vi "setStepNLoopParams.vi"(0 "Controller in":refnum<class "_Controller.lvclass">, 2 "axis (only applicable to multi-axis applications)":T3, 3 "set_params?":T2, 4 "step_n_params":T1, 5 "error in (no error)":errorcluster) -> (14 "Controller out":refnum<class "_Controller.lvclass">, 17 "success?":bool, 18 "response":string, 19 "error out":errorcluster)   [LabVIEW 2020, in "classes.lvlib" / "_Controller.lvclass"]
doc: "Use this VI to set the Step N Loop parameters to the referenced device at the specified index. For single axis applications, the axis input need not be specified.\n\nThere are two key cluster inputs to this VI: \"set_params?\" and \"set_n_params\". \n\n<B>step_n_params</B> allows the user to set the Step N Paramters if his/her choosing (minus the \"enabled\" status, which is handled via the Enable Step N Loop and Disable Step N Loop action VIs). \n<B>set_params?</B> contains boolean values that correspond to each settable parameter.\n\nIf the User wishes to only set the step_N_loop_ratio value to .75 while leaving all other parameters untouched, simply fill in the step_N_loop_ratio entry in the step_n_params cluster and set ONLY the \"set_ratio?\" boolean to TRUE in the \"set_params?' cluster.\n\nProduced By:\n\n<B>Kod Integrations, LLC</B>\n4835 Marianne Drive\nMount Airy, MD 21771\nhttp://www.kodintegrations.com\nemail: info@kodintegrations.com\nphone: (240) 687-1288"
uses:
  _Controller.lvclass
  common/controls/axis.ctl
  common/controls/step_n_loop_params_write_logic.ctl
  common/controls/step_n_params.ctl
  libraries/common.lvlib
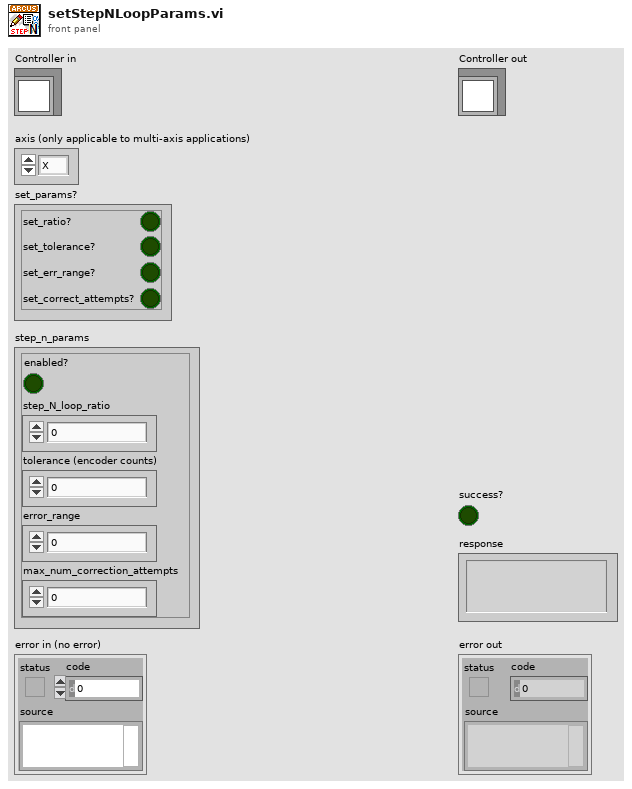
[diagram p1: front panel]
types:
  T1 = typedef "common.lvlib/step_n_params.ctl" = cluster{"step_N_loop_ratio":dbl, "tolerance (encoder counts)":u32, "error_range":i32, "max_num_correction_attempts":i32, "enabled?":bool}
  T2 = typedef "common.lvlib/step_n_loop_params_write_logic.ctl" = cluster{"set_ratio?":bool, "set_tolerance?":bool, "set_err_range?":bool, "set_correct_attempts?":bool}
  T3 = typedef "common.lvlib/axis.ctl" = enum16{"X", "Y", "Z", "U"}
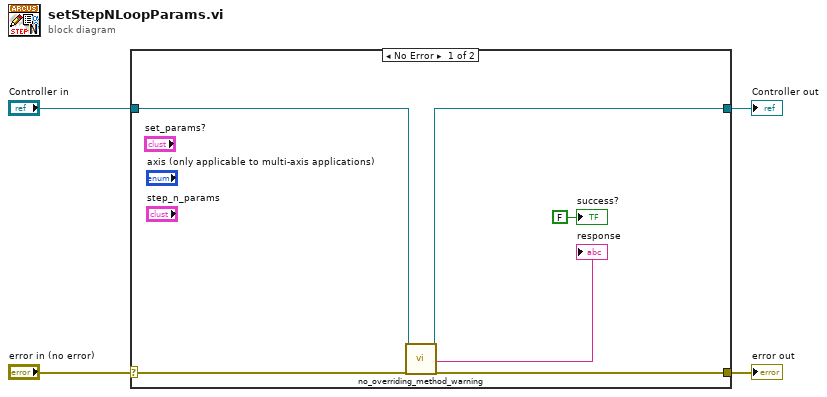
[diagram p0: block diagram]
diagram:
  n1 = case shown="No Error" "error in (no error)" {
    selector: "error in (no error)" -> [w10 w12]
    tunnel: [w9 w12] -> w3
    tunnel: [w7 w11] -> w1
    tunnel: "Controller in" -> [w8 w11]
    frame No Error {
      n2 = call "no_overriding_method_warning.vi"("Controller (in)"=w8, "error in (no error)"=w10) -> ("Controller (out)"=w7:refnum<class "_Controller.lvclass">, "msg"=→"response":string, "error out"=w9:errorcluster)  [unwired: 15 in]
      "success?" <- FALSE ("success?")
    }
    frame Error {
    }
  }
  "error out" <- w3
  "Controller out" <- w1
